vi "RunQDC_nice.vi"() -> ()   [LabVIEW 2014]
uses:
  <vilib>/addons/h5labview2/base/hid_t.ctl
  <vilib>/Utility/error.llb/DialogType.ctl
  Program Files (x86)/CAEN/Comm/labview/CAENComm.lvlib
  <vilib>/addons/h5labview2/file/H5F.lvlib
panel:
  out "error out":errorcluster
  out "Bottom Loop":i32
  out "Top loop":i32
  out "# Events Written":i32
  out "Current State":T1(ring)
  out "# Events Acquired (VME)":u32
  out "Processing\nErrors":errorcluster
  in  "# Events to\nRecord":i32
  in  "Low Range threshold":u16=1 min=1 max=4096
  in  "High range threshold":u16=32 min=1 max=4096
  in  "Count only accepted trigs?\n(else all trigs)":bool=TRUE
  in  "VME module Base Address":u32=4026793984 format="%.0x"
  in  "# of events before transfer":u16=1 min=1 max=32
  out "HDF5 File Handle":T2 format="%.0x"
  out "Acquisition\nErrors":errorcluster
  in  "STOP":bool
  in  "Stop Acquisition?":bool
  in  "Start Acquisition?":bool
  in  "Config File?":bool
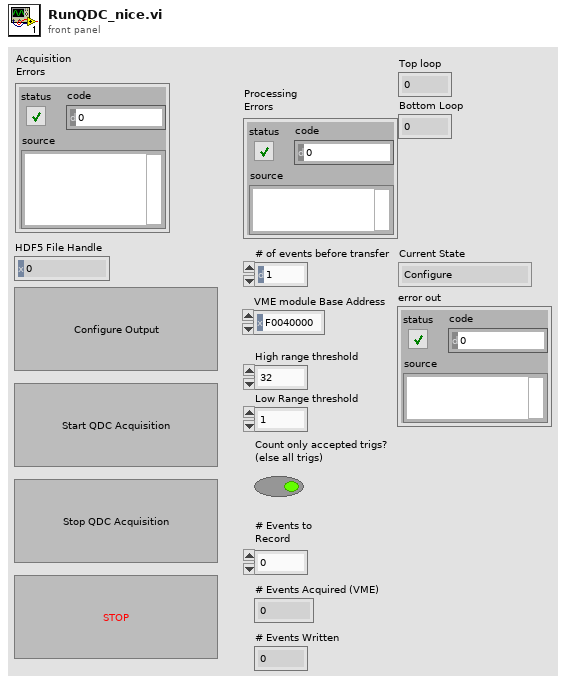
[diagram p1: front panel]
types:
  T1 = enum16{"Configure", "Initialise", "Run", "Close"}
  T2 = typedef "hid_t.ctl" = i32
  T3 = cluster{"State":enum16{"Startup", "Initialise", "Event OK", "Discard Event", "Exit", "Close"}, "Data":variant}
  T4 = enum16{"Startup", "Initialise", "Event OK", "Discard Event", "Exit", "Close"}
  T5 = typedef "DialogType.ctl" = u16
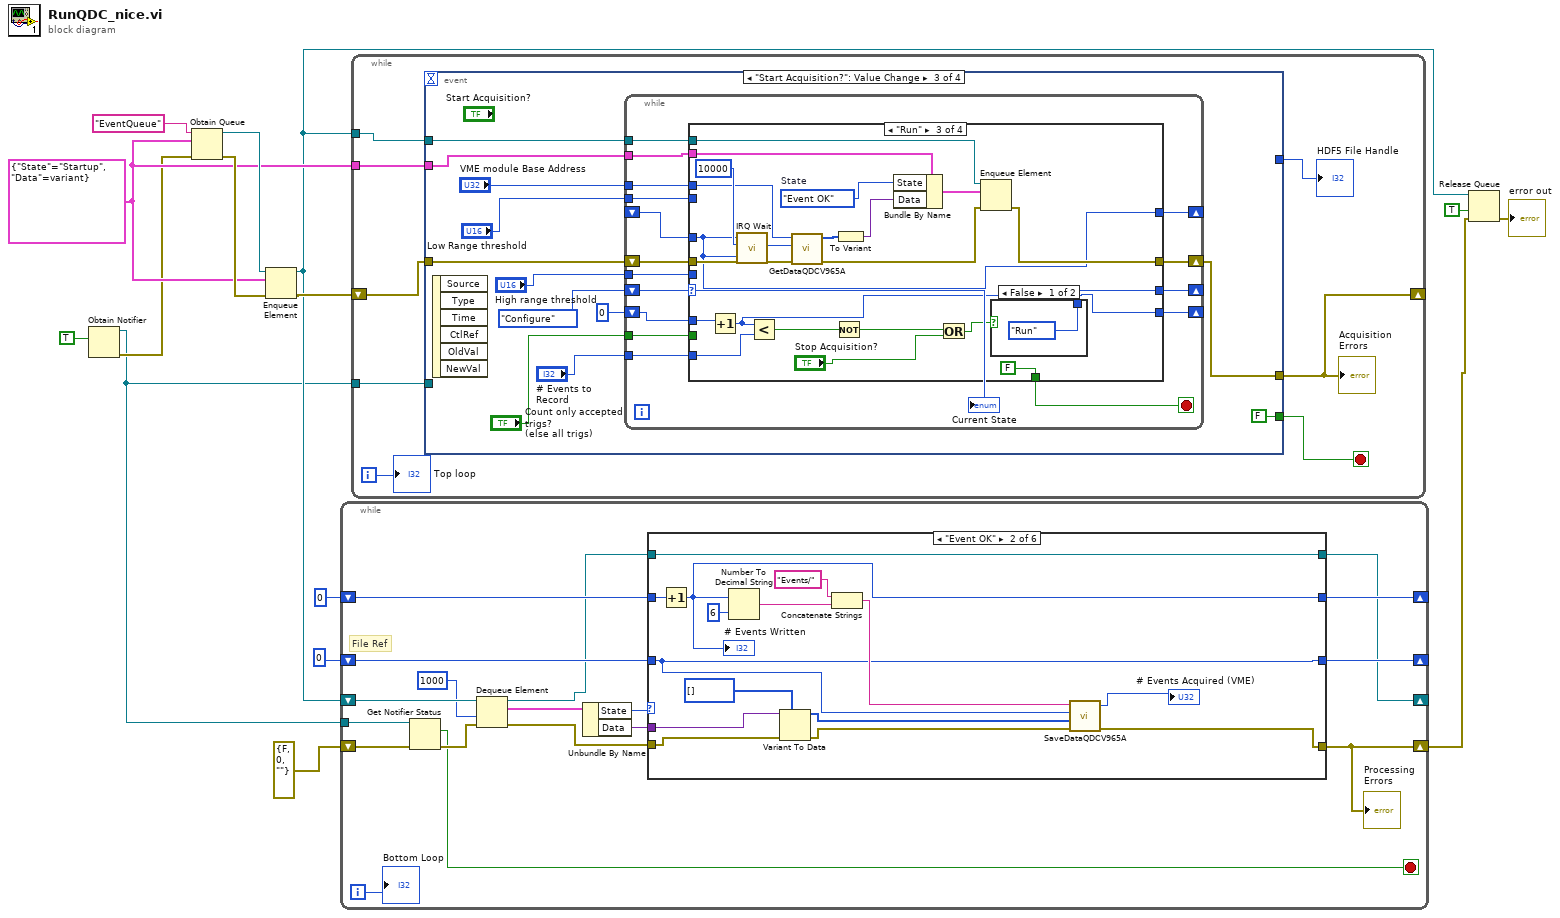
[diagram p0: block diagram]
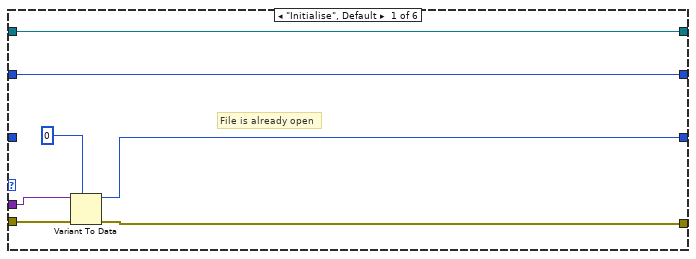
[diagram p2: hidden frame]
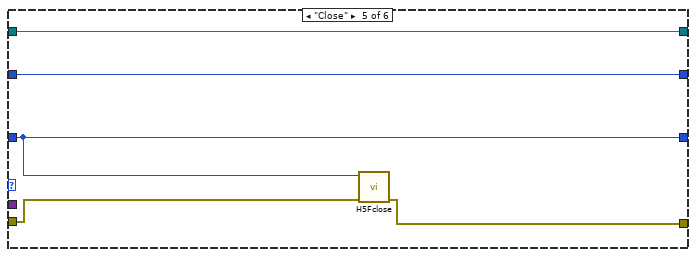
[diagram p5: hidden frame]
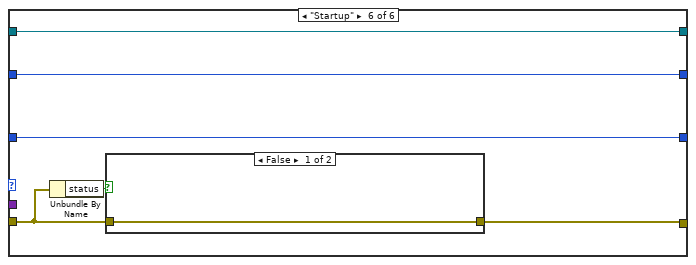
[diagram p6: hidden frame]
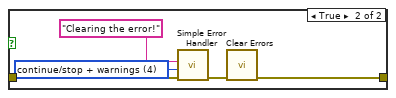
[diagram p7: hidden frame]
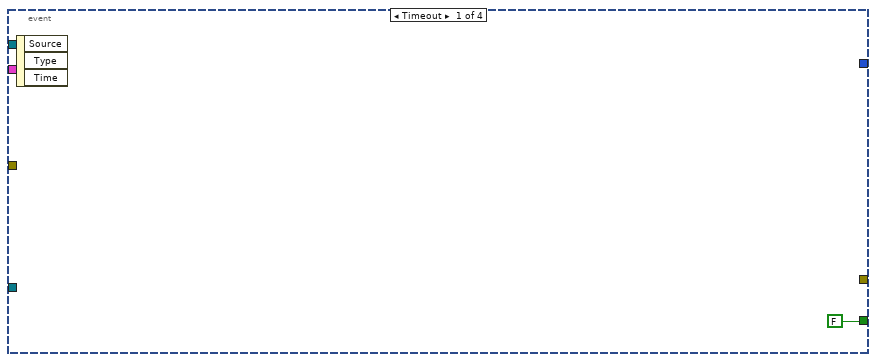
[diagram p8: hidden frame]
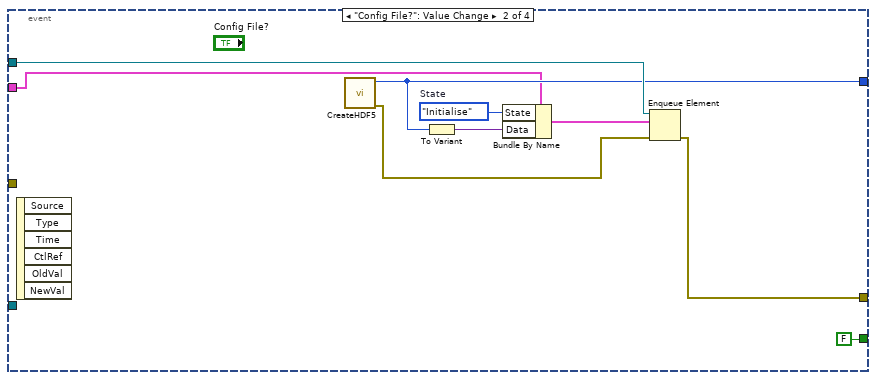
[diagram p9: hidden frame]
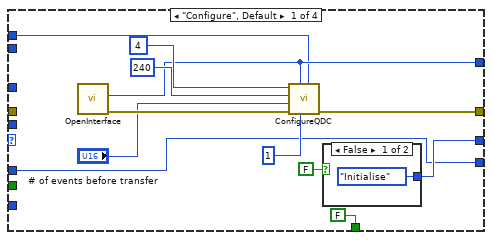
[diagram p10: hidden frame]
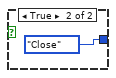
[diagram p11: hidden frame]
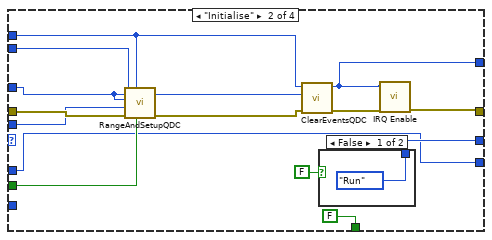
[diagram p12: hidden frame]
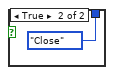
[diagram p13: hidden frame]
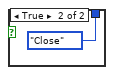
[diagram p14: hidden frame]
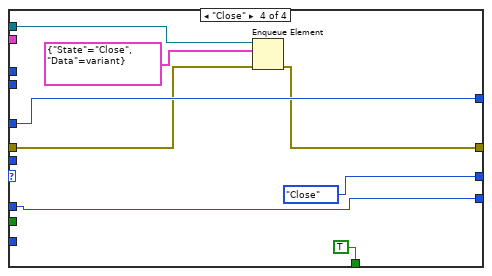
[diagram p15: hidden frame]
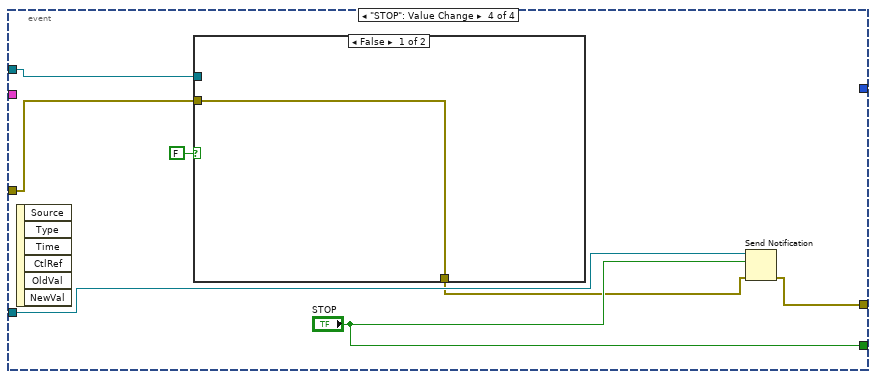
[diagram p16: hidden frame]
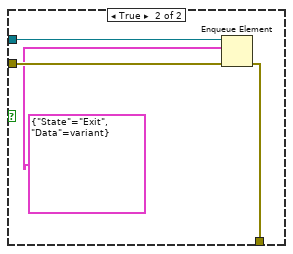
[diagram p17: hidden frame]
diagram:
  w11 = T3 {"State"=enum."Startup", "Data"=variant}
  n1 = Obtain Notifier(notification data type=TRUE) -> (notifier out=w4:refnum<notifier>, error out=w5:errorcluster)  [unwired: 3 in, 1 out]
  n2 = Obtain Queue(name (unnamed)="EventQueue", element data type=w11, error in (no error)=w5) -> (queue out=w12:refnum<queue>, error out=w13:errorcluster)  [unwired: 2 in, 1 out]
  n3 = Enqueue Element(queue=w12, element=w11, error in (no error)=w13) -> (queue out=w7:refnum<queue>, error out=w14:errorcluster)  [unwired: 1 in, 1 out]
  n4 = while {
    shift-right: [w28] -> _
    shift-left: w7 -> [w23]
    shift-right: [w30] -> w3
    shift-left: errorcluster {"status"=FALSE, "code"=0, "source"=""} ("error out") -> [w21]
    shift-right: [w33] -> _
    shift-left: T2 0 ("File Handle") -> [w32]
    shift-right: [w29] -> _
    shift-left: 0 -> [w31]
    tunnel: w4 -> [w19]
    i -> [w22]
    stop <- w17 stop-if-true
    # "File Ref"
    n5 = Get Notifier Status(notifier=w19, error in (no error)=w21) -> (current notification=w17:bool, error out=w20:errorcluster)  [unwired: 3 out]
    n6 = Dequeue Element(queue=w23, timeout in ms (-1)=1000, error in (no error)=w20) -> (queue out=w26:refnum<queue>, element=w27:T3, error out=w16:errorcluster)  [unwired: 1 out]
    n7 = Unbundle By Name(w27) -> ("State"=w24:T4, "Data"=w25:variant)
    n8 = case shown="\"Event OK\"" w24 {
      tunnel: [w39 w44 w59 w62 w67 w69] -> w30
      tunnel: w16 -> [w40 w48 w59 w62 w68 w70]
      tunnel: w25 -> [w38 w49 _ _ _ _]
      tunnel: [w36 w50 w58 w63 w66 w74] -> w33
      tunnel: w32 -> [_ w50 w58 w63 w66 w74]
      tunnel: w31 -> [w35 w55 w57 w61 w65 w73]
      tunnel: [w35 w43 w57 w61 w65 w73] -> w29
      tunnel: w26 -> [w34 w42 w56 w60 w64 w72]
      tunnel: [w34 w42 w56 w60 w64 w72] -> w28
      frame "Initialise", Default {
        # "File is already open"
        n9 = Variant To Data(error in=w40, type=T2 0 ("File Handle"), Variant=w38) -> (data=w36:T2, error out=w39:errorcluster)
      }
      frame "Event OK" {
        n10 = Increment(x=w55) -> (x+1=w43:i32)
        "# Events Written" <- w43
        n11 = Number To Decimal String(number=w43, width (-)=i16 6) -> (decimal integer string=w52:string)
        n12 = Variant To Data(error in=w48, type=u32[] [] ("Buff"), Variant=w49) -> (data=w45:u32[], error out=w47:errorcluster)
        n13 = Concatenate Strings("Events/", w52) -> (w51:string)
        n14 = call "SaveDataQDCV965A.vi"("error in (no error)"=w47, "Buff"=w45, "File Handle"=w50, "String"=w51) -> ("error out"=w44:errorcluster, "# Events Acquired (VME)"=→"# Events Acquired (VME)":u32)  [unwired: 6 in]
      }
      frame "Discard Event" {
      }
      frame "Exit" {
      }
      frame "Close" {
        n15 = call <vilib>:"H5Fclose.vi"("error in (no error)"=w68, "ref"=w66) -> ("error out"=w67:errorcluster)  [unwired: 9 in]
      }
      frame "Startup" {
        n16 = Unbundle By Name(w70) -> ("status"=w71:bool)
        n17 = case shown="False" w71 {
          tunnel: w70 -> [w75 w80]
          tunnel: [w75 w77] -> w69
          frame False {
          }
          frame True {
            w76 = T5 4 items=["no dialog", "OK message", "continue or stop message", "OK message + warnings", "continue/stop + warnings"] ("type of dialog (OK msg:1)")
            n18 = call <vilib>:"Simple Error Handler.vi"("error source (\" \")"="Clearing the error!" ("error source (\" \")"), "type of dialog (OK msg:1)"=w76, "error in (no error)"=w80) -> ("error out"=w78:errorcluster)  [unwired: 2 in, 4 out]
            n19 = call <vilib>:"Clear Errors.vi"("error in (no error)"=w78) -> ("error out"=w77:errorcluster)  [unwired: 5 in, 1 out]
          }
        }
      }
    }
    "Processing\nErrors" <- w30
    "Bottom Loop" <- w22
  }
  n20 = while {
    shift-right: [w86] -> _
    shift-left: w14 -> [w85]
    tunnel: w11 -> [w83]
    tunnel: w7 -> [w84]
    tunnel: w4 -> [w81]
    i -> [w82]
    stop <- w87 stop-if-true
    n21 = event shown="[2] \"Start Acquisition?\": Value Change" {
      selector: _ -> [_ _ _ _]
      dyn-events: _ -> [_ _ _ _]
      timeout: _ -> [_ _ _ _]
      tunnel: [_ w90 w109 w189] -> w86
      tunnel: [_ w96 _ _] -> w88
      tunnel: [FALSE FALSE FALSE ("STOP") "STOP"] -> w87
      tunnel: w85 -> [_ _ w108 w195]
      tunnel: w84 -> [_ w97 w101 w194]
      tunnel: w83 -> [_ w92 w100 _]
      tunnel: w81 -> [_ _ _ w192]
      event Timeout {
        n22 = event-data() -> ()  [unwired: 1 in, 3 out]
      }
      event "Config File?": Value Change {
        w95 = T4."Initialise"  # State
        n23 = event-data() -> ()  [unwired: 1 in, 6 out]
        n24 = call "CreateHDF5.vi"() -> ("error out"=w91:errorcluster, "File Handle"=w96:T2)  [unwired: 10 in]
        n25 = To Variant(anything=w96) -> (Variant=w94:variant)
        n26 = Bundle By Name(cluster=w92, "State"=w95, "Data"=w94) -> (w93:T3)
        n27 = Enqueue Element(queue=w97, element=w93, error in (no error)=w91) -> (error out=w90:errorcluster)  [unwired: 1 in, 2 out]
      }
      event "Start Acquisition?": Value Change {
        n28 = event-data() -> ()  [unwired: 1 in, 6 out]
        n29 = while {
          shift-right: [w117] -> _
          shift-left: T1."Configure" -> [w126]
          shift-right: [w125] -> w109
          shift-left: w108 -> [w123]
          shift-right: [w124] -> _
          shift-left: _ -> [w121]
          tunnel: "VME module Base Address" -> [w122]
          tunnel: "Count only accepted trigs?\n(else all trigs)" -> [w120]
          tunnel: "High range threshold" -> [w119]
          tunnel: "Low Range threshold" -> [w118]
          shift-right: [w113] -> _
          shift-left: 0 -> [w116]
          tunnel: "# Events to\nRecord" -> [w115]
          tunnel: w100 -> [w111]
          tunnel: w101 -> [w112]
          stop <- w114 stop-if-true
          n30 = case shown="\"Run\"" w126 {
            tunnel: [w133 w145 w163 w181] -> w125
            tunnel: [w132 w144 w157 w187] -> w124
            tunnel: w123 -> [_ w154 w178 w182]
            tunnel: w122 -> [w131 w148 w175 _]
            tunnel: w121 -> [_ w149 w157 w187]
            tunnel: w120 -> [_ w153 _ _]
            tunnel: w119 -> [_ w152 _ _]
            tunnel: w118 -> [_ w151 _ _]
            tunnel: [w130 w147 w174 T1."Close"] -> w117
            tunnel: w116 -> [w128 w142 w173 w185]
            tunnel: w115 -> [_ _ w172 _]
            tunnel: [FALSE FALSE FALSE TRUE] -> w114
            tunnel: [w128 w142 w169 w185] -> w113
            tunnel: w112 -> [_ _ w166 w184]
            tunnel: w111 -> [_ _ w168 _]
            frame "Configure", Default {
              n31 = call "OpenInterface.vi"() -> ("error out"=w138:errorcluster, "handle"=w132:i32)  [unwired: 9 in, 1 out]
              n32 = call "ConfigureQDC.vi"("VME module Base Address"=w131, "IRQ Lvl"=u16 1, "handle"=w132, "error in (no error)"=w138, "# of events before transfer (max 32)"="# of events before transfer", "CBLT Addr"=u16 240, "Geo Addr"=u16 4) -> ("error out"=w133:errorcluster)  [unwired: 3 in, 1 out]
              n33 = case shown="False" FALSE {
                tunnel: [T1."Initialise" T1."Close"] -> w130
                frame False {
                }
                frame True {
                }
              }
            }
            frame "Initialise" {
              n34 = call "RangeAndSetupQDC.vi"("Count only accepted trigs?\n(else all trigs)"=w153, "VME module Base Address"=w148, "error in (no error)"=w154, "High range threshold"=w152, "handle in"=w149, "Low Range threshold"=w151) -> ("error out"=w150:errorcluster)  [unwired: 4 in, 1 out]
              n35 = call "ClearEventsQDC.vi"("error in (no error)"=w150, "handle"=w149, "VME module Base Address"=w148) -> ("error out"=w146:errorcluster, "handle out"=w144:i32)  [unwired: 6 in, 1 out]
              n36 = case shown="False" FALSE {
                tunnel: [T1."Run" T1."Close"] -> w147
                frame False {
                }
                frame True {
                }
              }
              n37 = call "IRQ Enable.vi"("error in (no error)"=w146, "handle"=w144) -> ("error out"=w145:errorcluster)  [unwired: 9 in]
            }
            frame "Run" {
              w161 = T4."Event OK"  # State
              n38 = Increment(x=w173) -> (x+1=w169:i32)
              n39 = call "IRQ Wait.vi"("error in (no error)"=w178, "Timeout"=u32 10000, "handle"=w157) -> ("error out"=w176:errorcluster)  [unwired: 8 in]
              n40 = Less?(x=w169, y=w172) -> (x < y?=w160:bool)
              n41 = call "GetDataQDCV965A.vi"("error in (no error)"=w176, "handle in"=w157, "VME module Base Address"=w175) -> ("error out"=w165:errorcluster, "Data"=w162:u32[])  [unwired: 6 in, 1 out]
              n42 = Not(x=w160) -> (.not. x?=w159:bool)
              n43 = To Variant(anything=w162) -> (Variant=w167:variant)
              n44 = Bundle By Name(cluster=w168, "State"=w161, "Data"=w167) -> (w164:T3)
              n45 = Or(x=w159, y="Stop Acquisition?") -> (x .or. y?=w171:bool)
              n46 = Enqueue Element(queue=w166, element=w164, error in (no error)=w165) -> (error out=w163:errorcluster)  [unwired: 1 in, 2 out]
              n47 = case shown="False" w171 {
                tunnel: [T1."Run" T1."Close"] -> w174
                frame False {
                }
                frame True {
                }
              }
            }
            frame "Close" {
              n48 = Enqueue Element(queue=w184, element=T3 {"State"=enum."Close", "Data"=variant}, error in (no error)=w182) -> (error out=w181:errorcluster)  [unwired: 1 in, 2 out]
            }
          }
          "Current State" <- w126
        }
      }
      event "STOP": Value Change {
        n49 = event-data() -> ()  [unwired: 1 in, 6 out]
        n50 = case shown="False" FALSE {
          tunnel: w195 -> [w196 w200]
          tunnel: [w196 w199] -> w190
          tunnel: w194 -> [_ w198]
          frame False {
          }
          frame True {
            n51 = Enqueue Element(queue=w198, element=T3 {"State"=enum."Exit", "Data"=variant}, error in (no error)=w200) -> (error out=w199:errorcluster)  [unwired: 1 in, 2 out]
          }
        }
        n52 = Send Notification(notification="STOP", notifier=w192, error in (no error)=w190) -> (error out=w189:errorcluster)  [unwired: 1 out]
      }
    }
    "Acquisition\nErrors" <- w86
    "HDF5 File Handle" <- w88
    "Top loop" <- w82
  }
  n53 = Release Queue(queue=w7, force destroy? (F)=TRUE, error in (no error)=w3) -> (error out=→"error out":errorcluster)  [unwired: 2 out]
